vi "test.vi"() -> ()   [LabVIEW 2023]
uses:
  TCxxxx.lvlib
panel:
  out "Numeric":i32
  out "error IO":errorcluster
  out "String":string
  out "Return Count 2":u32
  out "Return Count":u32
  out "Read Buffer 10":string
  in  "Write Buffer 10":string="\u0015"
  out "Read Buffer 9":string
  out "Read Buffer 8":string
  out "Read Buffer 7":string
  in  "Write Buffer 9":string="0"
  in  "Write Buffer 8":string="0"
  in  "Write Buffer 7":string="1"
  out "Read Buffer 6":string
  in  "Write Buffer 6":string="_"
  out "Read Buffer 5":string
  out "Read Buffer 4":string
  in  "Write Buffer 5":string="0"
  in  "Write Buffer 4":string="_"
  out "Read Buffer 3":string
  in  "Write Buffer 3":string="w"
  out "Read Buffer 2":string
  in  "Write Buffer 2":string="_"
  in  "Write Buffer":string="**A"
  out "error out":errorcluster
  in  "VISA resource name":refnum<visa-resource-name>
  out "Read Buffer":string
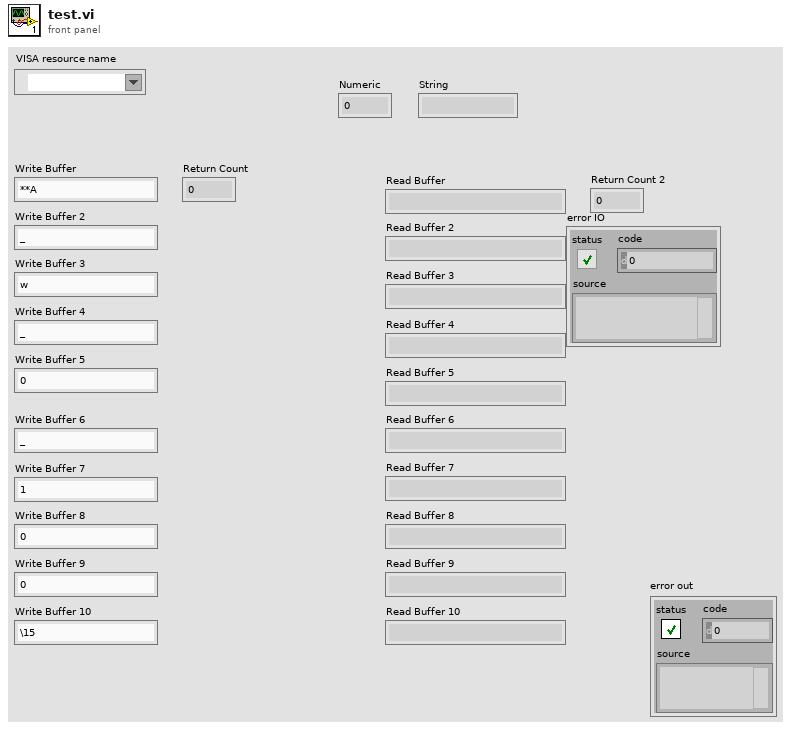
[diagram p1: front panel]
types:
  T1 = cluster{"Baud Rate":u32, "Parity":u16, "Data Bits":u16, "Stop Bits":u16, "Flow Control":u16}
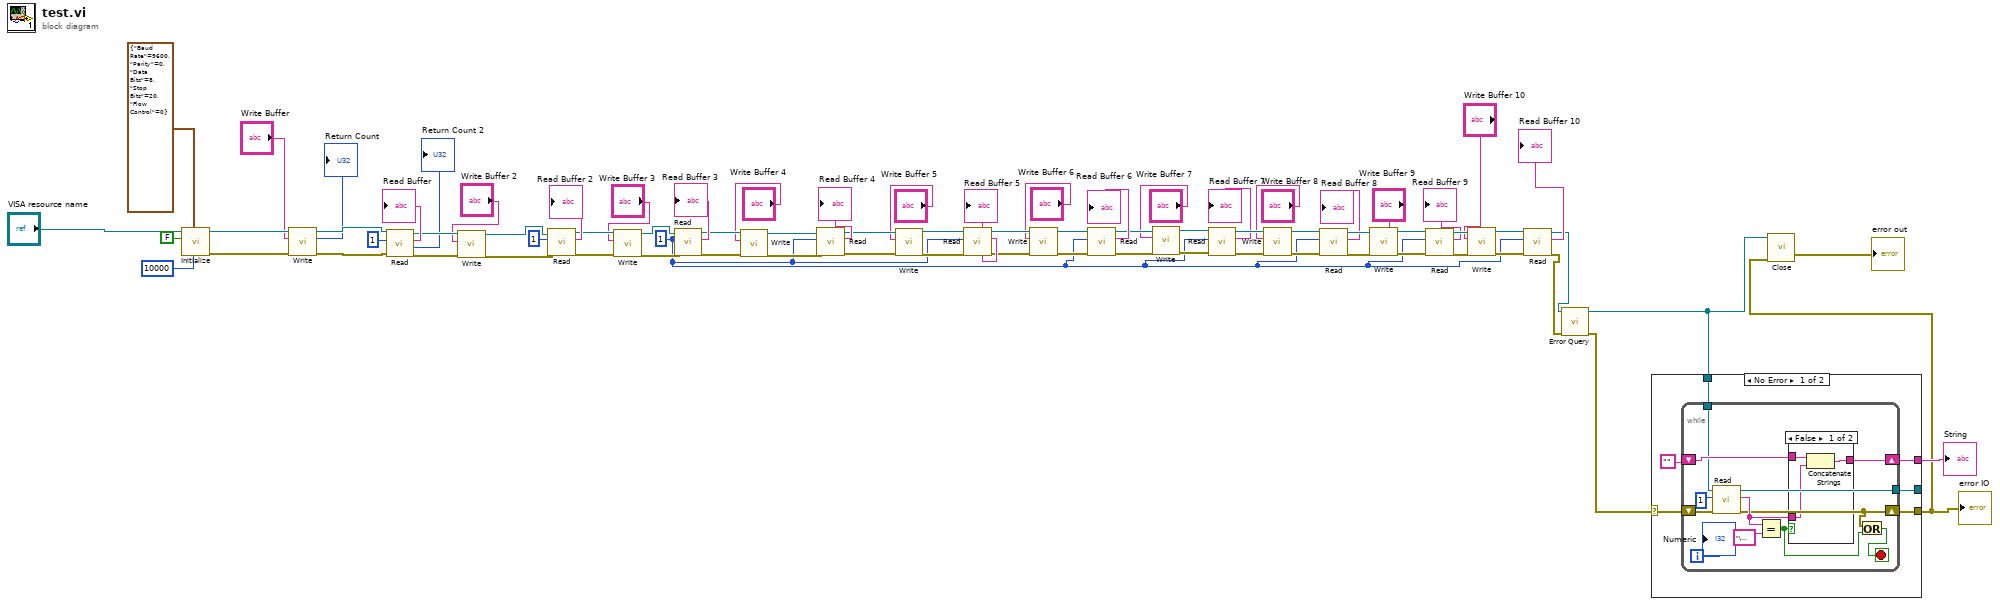
[diagram p0: block diagram]
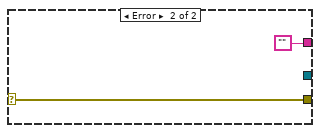
[diagram p3: hidden frame]
diagram:
  w7 = u32 1 ("Byte Count")
  n1 = call "Initialize.vi"("Timeout [ms]"=u32 10000, "Serial Configuration"=T1 {"Baud Rate"=9600, "Parity"=0, "Data Bits"=8, "Stop Bits"=20, "Flow Control"=0}, "ID Query (True)"=FALSE, "VISA resource name"="VISA resource name") -> ("error out"=w61:errorcluster, "VISA resource name out"=w64:refnum<visa-resource-name>)  [unwired: 6 in]
  n2 = call "Write.vi"("error in (no error)"=w61, "Write Buffer"="Write Buffer", "VISA resource name"=w64) -> ("error out"=w62:errorcluster, "Return Count"=→"Return Count":u32, "VISA resource name out"=w63:refnum<visa-resource-name>)  [unwired: 6 in]
  n3 = call "Read.vi"("error in (no error)"=w62, "Byte Count"=u32 1, "VISA resource name"=w63) -> ("error out"=w58:errorcluster, "Return Count"=→"Return Count 2":u32, "Read Buffer"=→"Read Buffer":string, "VISA resource name out"=w59:refnum<visa-resource-name>)  [unwired: 5 in]
  n4 = call "Write.vi"("error in (no error)"=w58, "Write Buffer"="Write Buffer 2", "VISA resource name"=w59) -> ("error out"=w55:errorcluster, "VISA resource name out"=w56:refnum<visa-resource-name>)  [unwired: 6 in, 1 out]
  n5 = call "Read.vi"("error in (no error)"=w55, "Byte Count"=u32 1, "VISA resource name"=w56) -> ("error out"=w53:errorcluster, "Read Buffer"=→"Read Buffer 2":string, "VISA resource name out"=w54:refnum<visa-resource-name>)  [unwired: 5 in, 1 out]
  n6 = call "Write.vi"("error in (no error)"=w53, "Write Buffer"="Write Buffer 3", "VISA resource name"=w54) -> ("error out"=w51:errorcluster, "VISA resource name out"=w52:refnum<visa-resource-name>)  [unwired: 6 in, 1 out]
  n7 = call "Read.vi"("error in (no error)"=w51, "Byte Count"=w7, "VISA resource name"=w52) -> ("error out"=w49:errorcluster, "Read Buffer"=→"Read Buffer 3":string, "VISA resource name out"=w46:refnum<visa-resource-name>)  [unwired: 5 in, 1 out]
  n8 = call "Write.vi"("error in (no error)"=w49, "Write Buffer"="Write Buffer 4", "VISA resource name"=w46) -> ("error out"=w48:errorcluster, "VISA resource name out"=w47:refnum<visa-resource-name>)  [unwired: 6 in, 1 out]
  n9 = call "Read.vi"("error in (no error)"=w48, "Byte Count"=w7, "VISA resource name"=w47) -> ("error out"=w44:errorcluster, "Read Buffer"=→"Read Buffer 4":string, "VISA resource name out"=w41:refnum<visa-resource-name>)  [unwired: 5 in, 1 out]
  n10 = call "Write.vi"("error in (no error)"=w44, "Write Buffer"="Write Buffer 5", "VISA resource name"=w41) -> ("error out"=w43:errorcluster, "VISA resource name out"=w42:refnum<visa-resource-name>)  [unwired: 6 in, 1 out]
  n11 = call "Read.vi"("error in (no error)"=w43, "Byte Count"=w7, "VISA resource name"=w42) -> ("error out"=w38:errorcluster, "Read Buffer"=→"Read Buffer 5":string, "VISA resource name out"=w39:refnum<visa-resource-name>)  [unwired: 5 in, 1 out]
  n12 = call "Write.vi"("error in (no error)"=w38, "Write Buffer"="Write Buffer 6", "VISA resource name"=w39) -> ("error out"=w36:errorcluster, "VISA resource name out"=w37:refnum<visa-resource-name>)  [unwired: 6 in, 1 out]
  n13 = call "Read.vi"("error in (no error)"=w36, "Byte Count"=w7, "VISA resource name"=w37) -> ("error out"=w29:errorcluster, "Read Buffer"=→"Read Buffer 6":string, "VISA resource name out"=w33:refnum<visa-resource-name>)  [unwired: 5 in, 1 out]
  n14 = call "Write.vi"("error in (no error)"=w29, "Write Buffer"="Write Buffer 7", "VISA resource name"=w33) -> ("error out"=w28:errorcluster, "VISA resource name out"=w32:refnum<visa-resource-name>)  [unwired: 6 in, 1 out]
  n15 = call "Read.vi"("error in (no error)"=w28, "Byte Count"=w7, "VISA resource name"=w32) -> ("error out"=w27:errorcluster, "Read Buffer"=→"Read Buffer 7":string, "VISA resource name out"=w31:refnum<visa-resource-name>)  [unwired: 5 in, 1 out]
  n16 = call "Write.vi"("error in (no error)"=w27, "Write Buffer"="Write Buffer 8", "VISA resource name"=w31) -> ("error out"=w26:errorcluster, "VISA resource name out"=w30:refnum<visa-resource-name>)  [unwired: 6 in, 1 out]
  n17 = call "Read.vi"("error in (no error)"=w26, "Byte Count"=w7, "VISA resource name"=w30) -> ("error out"=w24:errorcluster, "Read Buffer"=→"Read Buffer 8":string, "VISA resource name out"=w23:refnum<visa-resource-name>)  [unwired: 5 in, 1 out]
  n18 = call "Write.vi"("error in (no error)"=w24, "Write Buffer"="Write Buffer 9", "VISA resource name"=w23) -> ("error out"=w25:errorcluster, "VISA resource name out"=w22:refnum<visa-resource-name>)  [unwired: 6 in, 1 out]
  n19 = call "Read.vi"("error in (no error)"=w25, "Byte Count"=w7, "VISA resource name"=w22) -> ("error out"=w18:errorcluster, "Read Buffer"=→"Read Buffer 9":string, "VISA resource name out"=w19:refnum<visa-resource-name>)  [unwired: 5 in, 1 out]
  n20 = call "Write.vi"("error in (no error)"=w18, "Write Buffer"="Write Buffer 10", "VISA resource name"=w19) -> ("error out"=w20:errorcluster, "VISA resource name out"=w21:refnum<visa-resource-name>)  [unwired: 6 in, 1 out]
  n21 = call "Read.vi"("error in (no error)"=w20, "Byte Count"=w7, "VISA resource name"=w21) -> ("error out"=w2:errorcluster, "Read Buffer"=→"Read Buffer 10":string, "VISA resource name out"=w4:refnum<visa-resource-name>)  [unwired: 5 in, 1 out]
  n22 = call "Error Query.vi"("error in (no error)"=w2, "VISA resource name"=w4) -> ("error out"=w1:errorcluster, "VISA resource name out"=w3:refnum<visa-resource-name>)  [unwired: 8 in]
  n23 = case shown="No Error" w1 {
    selector: w1 -> [w82 w99]
    tunnel: [w80 ""] -> w6
    tunnel: [w79 w99] -> w5
    tunnel: [w78 _] -> _
    tunnel: w3 -> [w77 _]
    frame No Error {
      n24 = while {
        shift-right: [w88] -> w80
        shift-left: "" -> [w89]
        tunnel: [w91] -> w78
        tunnel: w77 -> [w87]
        shift-right: [w85] -> w79
        shift-left: w82 -> [w92]
        i -> [w86]
        stop <- w83 stop-if-true
        n25 = call "Read.vi"("error in (no error)"=w92, "Byte Count"=1, "VISA resource name"=w87) -> ("error out"=w85:errorcluster, "Read Buffer"=w90:string, "VISA resource name out"=w91:refnum<visa-resource-name>)  [unwired: 5 in, 1 out]
        n26 = Equal?(x=w90, y="\u0015") -> (x = y?=w84:bool)
        n27 = case shown="False" w84 {
          tunnel: w90 -> [w95 _]
          tunnel: w89 -> [w97 w98]
          tunnel: [w96 w98] -> w88
          frame False {
            n28 = Concatenate Strings(w97, w95) -> (w96:string)
          }
          frame True {
          }
        }
        n29 = Or(x=w85, y=w84) -> (x .or. y?=w83:bool)
        "Numeric" <- w86
      }
    }
    frame Error {
    }
  }
  "String" <- w6
  "error IO" <- w5
  n30 = call "Close.vi"("error in (no error)"=w5, "VISA resource name"=w3) -> ("error out"=→"error out":errorcluster)  [unwired: 9 in]
